vi "System@CounterReset__Parameter.vi"(1 "ParamterIn":string) -> (0 "ParamterOut":string)   [LabVIEW 2019]
panel:
  in  "Number":string(combo)
  in  "Counter":string(combo)
  in  "Confirm":bool
  # "System@CounterReset $Counter,$Number"
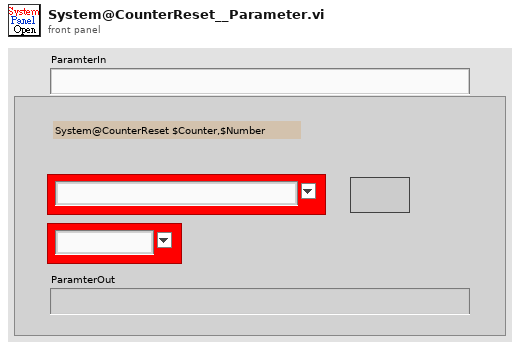
[diagram p1: front panel]
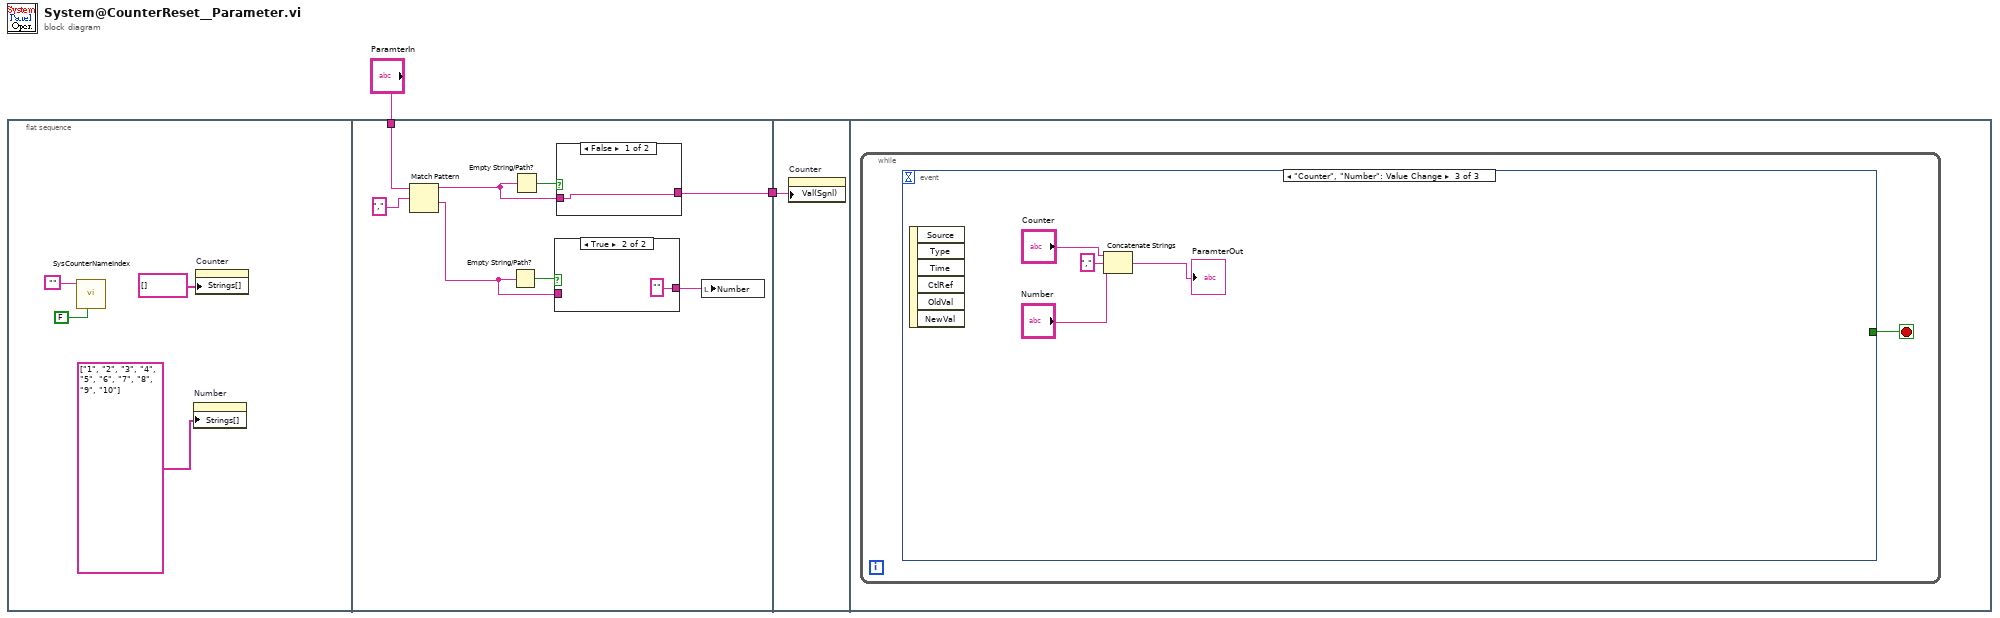
[diagram p0: block diagram]
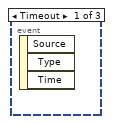
[diagram p4: hidden frame]
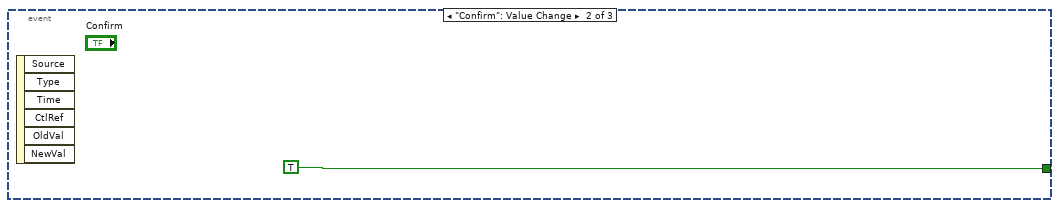
[diagram p5: hidden frame]
diagram:
  n1 = flat-sequence {
    tunnel: "ParamterIn" -> [w13]
    tunnel: [w8] -> w1
    tunnel: w1 -> [w19]
    frame #0 {
      n2 = call "SysCounterNameIndex.vi"("Reset"=FALSE, "Counter"="") -> ()  [unwired: 8 in, 2 out]
      n3 = property on="Number" class="CmbBox"("Strings[]"=string[] ["1", "2", "3", "4", "5", "6", "7", "8", "9", "10"] ("Strings []")) -> ()  [unwired: 2 in, 2 out]
      n4 = property on="Counter" class="CmbBox"("Strings[]"=string[] [] ("Strings []")) -> ()  [unwired: 2 in, 2 out]
    }
    frame #1 {
      n5 = Match Pattern(string=w13, regular expression=",") -> (before substring=w11:string, after substring=w9:string)  [unwired: 1 in, 2 out]
      n6 = Empty String/Path?(string/path=w9) -> (empty?=w10:bool)
      n7 = Empty String/Path?(string/path=w11) -> (empty?=w14:bool)
      n8 = case shown="True" w10 {
        tunnel: w9 -> [w15 _]
        tunnel: [w15 "" ("ParamterIn")] -> w7
        frame False {
        }
        frame True {
        }
      }
      n9 = case shown="False" w14 {
        tunnel: w11 -> [w17 w18]
        tunnel: [w17 w18] -> w8
        frame False {
        }
        frame True {
        }
      }
      n10 = local write "Number"(w7) -> ()
    }
    frame #2 {
      n11 = property on="Counter" class="CmbBox"("Val(Sgnl)"=w19) -> ()  [unwired: 2 in, 2 out]
    }
    frame #3 {
      n12 = while {
        stop <- w20 stop-if-true
        n13 = event shown="[2] \"Counter\", \"Number\": Value Change" {
          selector: _ -> [_ _ _]
          dyn-events: _ -> [_ _ _]
          timeout: _ -> [_ _ _]
          tunnel: [_ TRUE _] -> w20
          event Timeout {
            n14 = event-data() -> ()  [unwired: 1 in, 3 out]
          }
          event "Confirm": Value Change {
            n15 = event-data() -> ()  [unwired: 1 in, 6 out]
          }
          event "Counter", "Number": Value Change {
            n16 = event-data() -> ()  [unwired: 1 in, 6 out]
            n17 = Concatenate Strings("Counter", "," ("string"), "Number") -> (→"ParamterOut":string)
          }
        }
      }
    }
  }
